vi "CloseClaw.vi"(8 "error in":errorcluster, 9 "FPGA VI Reference In":refnum<k20>, 10 "milliseconds to wait \nfor servo to change":u32=100, 11 "Old Angle":dbl) -> (0 "error out":errorcluster, 1 "FPGA VI Reference Out":refnum<k20>, 2 "milliseconds to wait \nfor servo to change out":u32, 3 "New Angle":dbl)   [LabVIEW 2012]
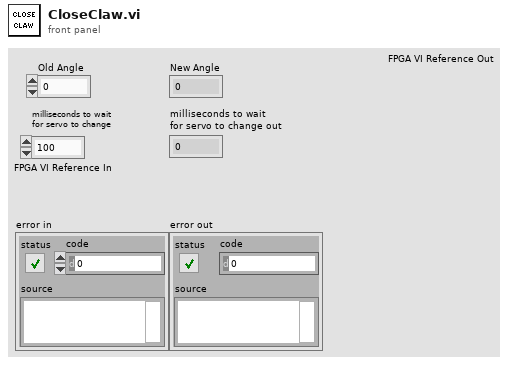
[diagram p1: front panel]
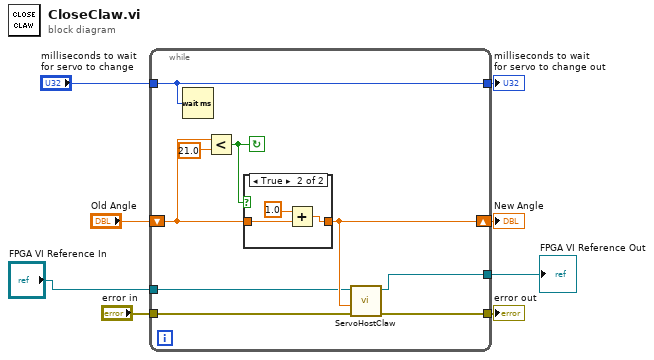
[diagram p0: block diagram]
diagram:
  n1 = while {
    tunnel: "error in" -> [w11]
    shift-right: [w12] -> w4
    shift-left: "Old Angle" -> [w15]
    tunnel: "milliseconds to wait \nfor servo to change" -> [w14]
    tunnel: [w13] -> w5
    tunnel: [w14] -> w3
    tunnel: "FPGA VI Reference In" -> [w10]
    tunnel: [w9] -> w1
    stop <- w16 continue-if-true
    n2 = Wait (ms)(milliseconds to wait=w14) -> ()  [unwired: 1 out]
    n3 = Less?(x=w15, y=21.0) -> (x < y?=w16:bool)
    n4 = case shown="True" w16 {
      tunnel: w15 -> [w18 w20]
      tunnel: [w18 w19] -> w12
      frame False {
      }
      frame True {
        n5 = Add(x=1.0, y=w20) -> (x+y=w19:dbl)
      }
    }
    n6 = call "ServoHostClaw.vi"("error in"=w11, "Angle (deg) Claw"=w12, "FPGA VI Reference In"=w10) -> ("error out"=w13:errorcluster, "FPGA VI Reference Out"=w9:refnum<k20>)  [unwired: 7 in]
  }
  "error out" <- w5
  "New Angle" <- w4
  "milliseconds to wait \nfor servo to change out" <- w3
  "FPGA VI Reference Out" <- w1
